vi "Sort.vi"(4 "Array":dbl[](array[numeric])) -> (0 "Indices":i32[](array[numeric]), 1 "Sorted array":dbl[](array[numeric]))   [LabVIEW 2009]
panel:
  # "Guillaume Plateau - yguig2@yahoo.fr"
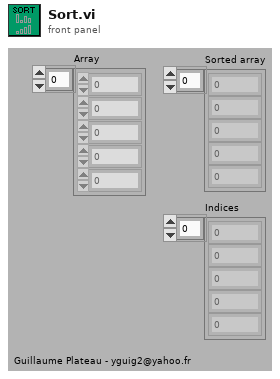
[diagram p1: front panel]
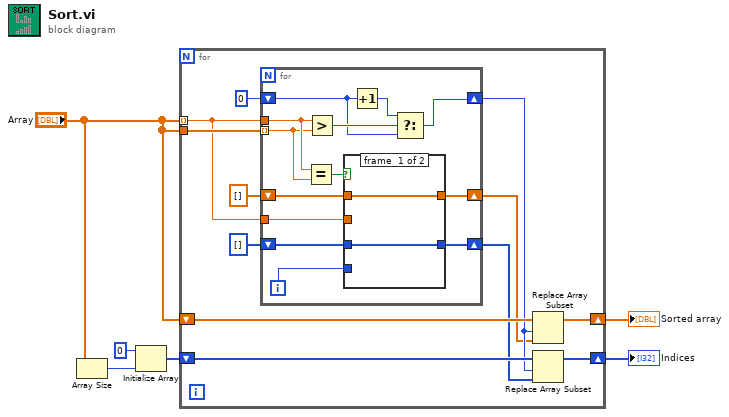
[diagram p0: block diagram]
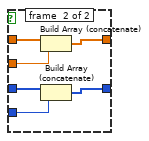
[diagram p2: hidden frame]
diagram:
  n1 = Array Size(array="Array") -> (size(s)=w4:i32)
  n2 = Initialize Array(0 ("element"), w4) -> (w3:i32[])
  n3 = for {
    tunnel: "Array" -> [w14] mode=indexing
    tunnel: "Array" -> [w18]
    shift-right: [w8] -> w6
    shift-left: "Array" -> [w13]
    shift-right: [w7] -> w5
    shift-left: w3 -> [w12]
    n4 = for {
      tunnel: w18 -> [w30] mode=indexing
      tunnel: w14 -> [w31]
      shift-right: [w25] -> w11
      shift-left: 0 -> [w27]
      shift-right: [w22] -> w10
      shift-left: dbl[] [] -> [w24]
      tunnel: w14 -> [w23]
      shift-right: [w21] -> w9
      shift-left: i32[] [] -> [w20]
      i -> [w19]
      n5 = Equal?(x=w31, y=w30) -> (x = y?=w29:bool)
      n6 = Greater?(x=w31, y=w30) -> (0:w28:bool)
      n7 = case shown="True" w29 {
        tunnel: w24 -> [w33 w39]
        tunnel: w23 -> [_ w38]
        tunnel: [w33 w37] -> w22
        tunnel: w20 -> [w32 w34]
        tunnel: w19 -> [_ w35]
        tunnel: [w32 w36] -> w21
        frame #0 {
        }
        frame #1 {
          n8 = Build Array (concatenate)(w39, w38) -> (w37:dbl[])
          n9 = Build Array (concatenate)(w34, w35) -> (w36:i32[])
        }
      }
      n10 = Increment(x=w27) -> (x+1=w26:i32)
      n11 = Select(t=w26, s=w28, f=w27) -> (s? t:f=w25:i32)
    }
    n12 = Replace Array Subset(array=w13, new element=w10, index=w11) -> (w8:dbl[])
    n13 = Replace Array Subset(array=w12, new element=w9, index=w11) -> (w7:i32[])
  }
  "Sorted array" <- w6
  "Indices" <- w5
